vi "Program ILC.vi"(0 "Model in":refnum<class "Model.lvclass">, 11 "error in (no error)":errorcluster) -> (4 "Model out":refnum<class "Model.lvclass">, 15 "error out":errorcluster)   [LabVIEW 2016, in "Model.lvclass"]
uses:
  Model.lvclass
  Model.lvclass/Model.ctl
  Modbus/DesktopModbus/DesktopModbus.lvclass
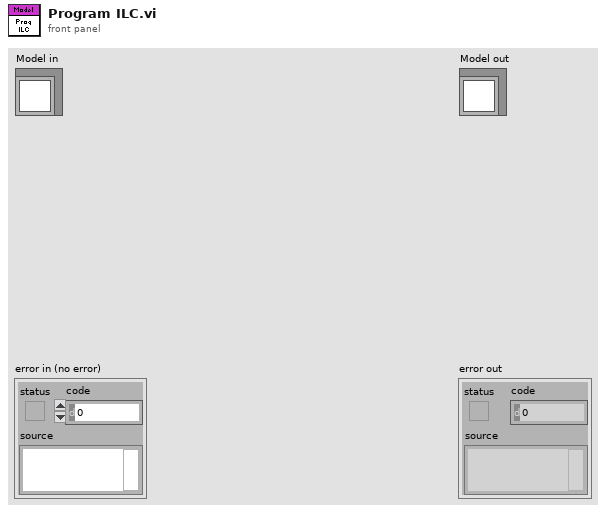
[diagram p1: front panel]
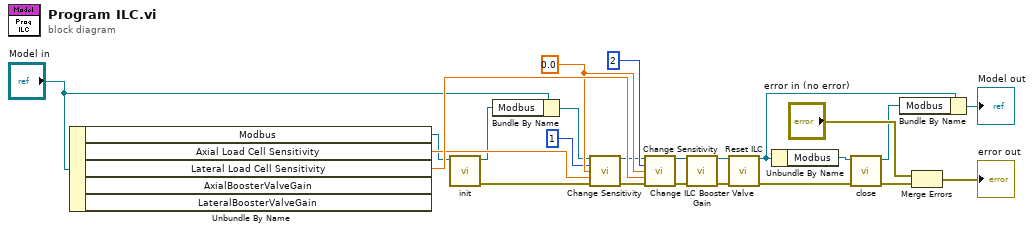
[diagram p0: block diagram]
diagram:
  w22 = sgl 0.0 ("Offset")
  n1 = Unbundle By Name("Model in") -> ("Modbus"=w17:refnum<class "DesktopModbus.lvclass">, "Axial Load Cell Sensitivity"=w19:dbl, "Lateral Load Cell Sensitivity"=w23:dbl)  [unwired: 2 out]
  n2 = call "init.vi"("DesktopModbus in"=w17) -> ("error out"=w7:errorcluster, "DesktopModbus out"=w13:refnum<class "DesktopModbus.lvclass">)  [unwired: 9 in]
  n3 = Bundle By Name(cluster="Model in", "Modbus"=w13) -> (w8:refnum<class "Model.lvclass">)
  n4 = call "Change Sensitivity.vi"("Model in"=w8, "Channel"=u8 1, "Offset"=w22, "Sensitivity"=w19, "error in (no error)"=w7) -> ("Model out"=w20:refnum<class "Model.lvclass">, "error out"=w24:errorcluster)  [unwired: 9 in]
  n5 = call "Change Sensitivity.vi"("Model in"=w20, "Channel"=u8 2, "Offset"=w22, "Sensitivity"=w23, "error in (no error)"=w24) -> ("Model out"=w4:refnum<class "Model.lvclass">, "error out"=w1:errorcluster)  [unwired: 9 in]
  n6 = call "Change ILC Booster Valve Gain.vi"("Model in"=w4, "error in (no error)"=w1) -> ("Model out"=w3:refnum<class "Model.lvclass">, "error out"=w2:errorcluster)  [unwired: 12 in]
  n7 = call "Reset ILC.vi"("Model in"=w3, "error in (no error)"=w2) -> ("Model out"=w6:refnum<class "Model.lvclass">, "error out"=w5:errorcluster)  [unwired: 12 in]
  n8 = Unbundle By Name(w6) -> ("Modbus"=w12:refnum<class "DesktopModbus.lvclass">)
  n9 = call "close.vi"("error in (no error)"=w5, "DesktopModbus in"=w12) -> ("error out"=w9:errorcluster, "DesktopModbus out"=w11:refnum<class "DesktopModbus.lvclass">)  [unwired: 8 in]
  n10 = Bundle By Name(cluster=w6, "Modbus"=w11) -> (→"Model out":refnum<class "Model.lvclass">)
  n11 = Merge Errors("error in (no error)", w9) -> (→"error out":errorcluster)
